vi "Set Cell (String).vi"(6 "Column":i32, 7 "Value":string, 8 "error in (no error)":errorcluster, 9 "Row":i32, 10 "Sheet Reference":refnum<k24>) -> (0 "error out":errorcluster, 2 "Sheet Reference out":refnum<k24>)   [LabVIEW 2014]
uses:
  C:/Users/LENOVO/Desktop/CodeSpace GUI/LVExcel/Resources/net40/NPOI.dll
  Resources/net40/NPOI.dll
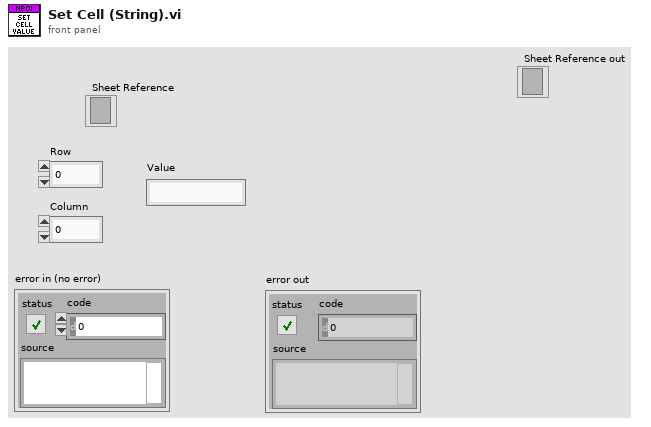
[diagram p1: front panel]
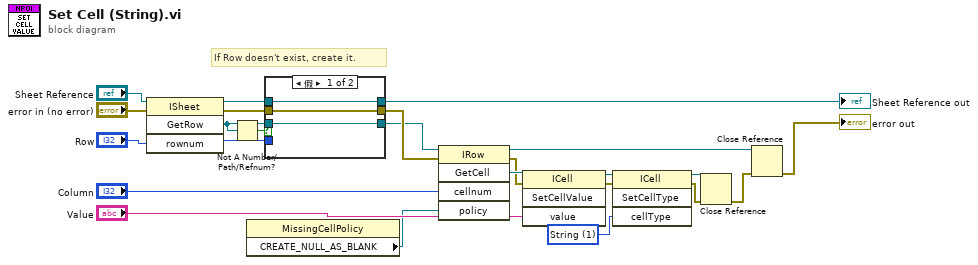
[diagram p0: block diagram]
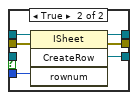
[diagram p2: hidden frame]
diagram:
  w1 = 1 items=["Numeric"=0, "String"=1, "Formula"=2, "Blank"=3, "Boolean"=4, "Error"=5, "Unknown"=-1] ("cellType")
  # "If Row doesn't exist, create it."
  n1 = invoke class="ISheet" method="GetRow"(reference="Sheet Reference", error in="error in (no error)", "rownum"="Row") -> (reference out=w12:refnum<k24>, error out=w13:errorcluster, "GetRow"=w15:refnum<k24>)  [unwired: 1 in, 1 out]
  n2 = Not A Number/Path/Refnum?(number/path/refnum=w15) -> (NaN/Path/Refnum?=w14:bool)
  n3 = property class="MissingCellPolicy"() -> ("CREATE_NULL_AS_BLANK"=w5:refnum<k24>)  [unwired: 2 in, 2 out]
  n4 = case shown="假" w14 {
    tunnel: w12 -> [w26 w32]
    tunnel: w13 -> [w25 w31]
    tunnel: [w25 w30] -> w7
    tunnel: [w26 w29] -> w8
    tunnel: "Row" -> [_ w28]
    tunnel: [w24 w27] -> w6
    tunnel: w15 -> [w24 _]
    frame False {
    }
    frame True {
      n5 = invoke class="ISheet" method="CreateRow"(reference=w32, error in=w31, "rownum"=w28) -> (reference out=w29:refnum<k24>, error out=w30:errorcluster, "CreateRow"=w27:refnum<k24>)  [unwired: 1 in, 1 out]
    }
  }
  "Sheet Reference out" <- w8
  n6 = invoke class="IRow" method="GetCell"(reference=w6, error in=w7, "cellnum"="Column", "policy"=w5) -> (reference out=w23:refnum<k24>, error out=w20:errorcluster, "GetCell"=w21:refnum<k24>)  [unwired: 1 in, 2 out]
  n7 = invoke class="ICell" method="SetCellValue"(reference=w21, error in=w20, "value"="Value") -> (reference out=w3:refnum<k24>, error out=w19:errorcluster)  [unwired: 1 in, 2 out]
  n8 = invoke class="ICell" method="SetCellType"(reference=w3, error in=w19, "cellType"=w1) -> (reference out=w2:refnum<k24>, error out=w4:errorcluster)  [unwired: 1 in, 2 out]
  n9 = Close Reference(reference=w2, error in (no error)=w4) -> (error out=w18:errorcluster)
  n10 = Close Reference(reference=w23, error in (no error)=w18) -> (error out=→"error out":errorcluster)
